vi "json head.vi"(11 "information":string[](array[string])=["@uutName@", "@uutCode@", "@SN@", "@computerName@", "@softName@", "@softVersion@", "@startTime@", "@stopTime@", "@result@"]) -> (3 "midVar_Content":string)   [LabVIEW 2011]
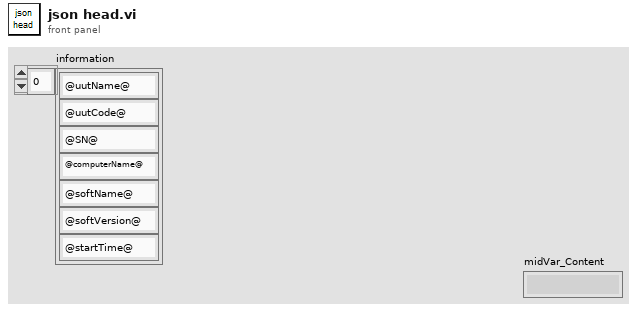
[diagram p1: front panel]
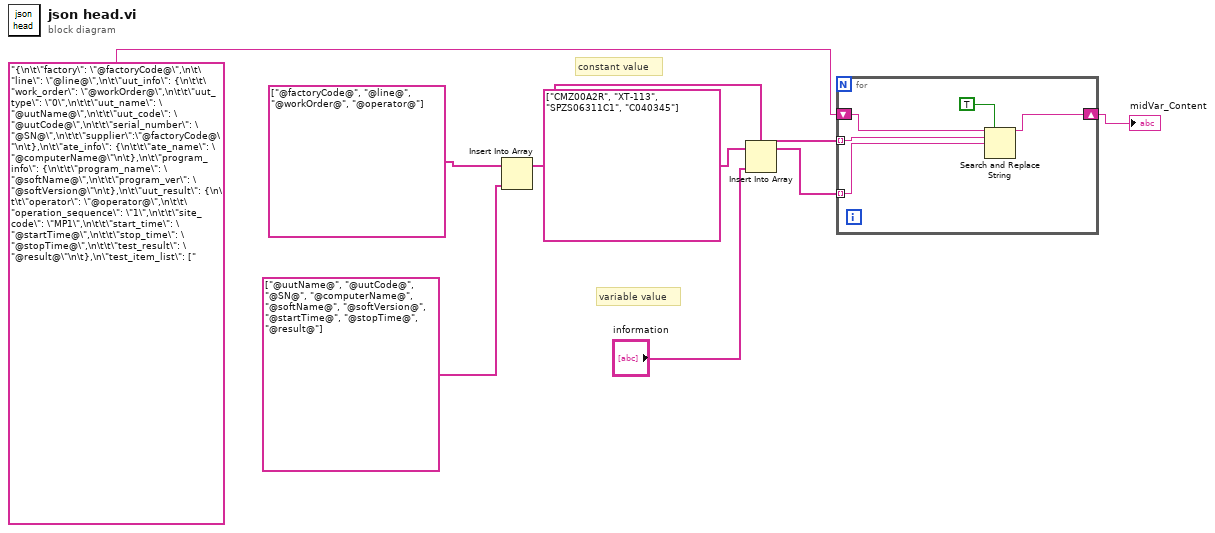
[diagram p0: block diagram]
diagram:
  # "variable value"
  # "constant value"
  n1 = Insert Into Array(array=string[] ["@factoryCode@", "@line@", "@workOrder@", "@operator@"], new element=string[] ["@uutName@", "@uutCode@", "@SN@", "@computerName@", "@softName@", "@softVersion@", "@startTime@", "@stopTime@", "@result@"]) -> (w4:string[])  [unwired: 1 in]
  n2 = Insert Into Array(array=string[] ["CMZ00A2R", "XT-113", "SPZS06311C1", "C040345"], new element="information") -> (w3:string[])  [unwired: 1 in]
  n3 = for {
    tunnel: w4 -> [w12] mode=indexing
    tunnel: w3 -> [w10] mode=indexing
    shift-right: [w9] -> w1
    shift-left: "{\n\t\"factory\": \"@factoryCode@\",\n\t\"line\": \"@line@\",\n\t\"uut_info\": {\n\t\t\"work_order\": \"@workOrder@\",\n\t\t\"uut_type\": \"0\",\n\t\t\"uut_name\": \"@uutName@\",\n\t\t\"uut_code\": \"@uutCode@\",\n\t\t\"serial_number\": \"@SN@\",\n\t\t\"supplier\":\"@factoryCode@\"\n\t},\n\t\"ate_info\": {\n\t\t\"ate_name\": \"@computerName@\"\n\t},\n\t\"program_info\": {\n\t\t\"program_name\": \"@softName@\",\n\t\t\"program_ver\": \"@softVersion@\"\n\t},\n\t\"uut_result\": {\n\t\t\"operator\": \"@operator@\",\n\t\t\"operation_sequence\": \"1\",\n\t\t\"site_code\": \"MP1\",\n\t\t\"start_time\": \"@startTime@\",\n\t\t\"stop_time\": \"@stopTime@\",\n\t\t\"test_result\": \"@result@\"\n\t},\n\"test_item_list\": [" -> [w13]
    n4 = Search and Replace String(replace all?=TRUE ("替换全部？(F)"), input string=w13, search string=w12, replace string=w10) -> (result string=w9:string)  [unwired: 4 in, 3 out]
  }
  "midVar_Content" <- w1
